vi "Shared Variable Creation.vi"() -> ()   [LabVIEW 2011]
uses:
  <vilib>/lvdsc/NI_DSC.lvlib
panel:
  out "error out 4":errorcluster
  out "error out 3":errorcluster
  out "error out 2":errorcluster
  out "error out":errorcluster
  out "process name out":string
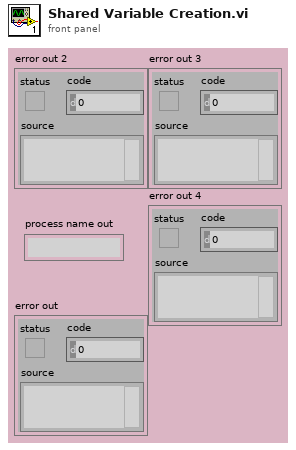
[diagram p1: front panel]
types:
  T1 = enum32{"u32BitField", "bool", "double", "string", "int8", "uint8", "int16", "uint16", "int32", "uint32", "int64", "uint64", "single", "double waveform", "int16 waveform", "array of boolean", "array of int8", "array of uint8", "array of int16", "array of uint16", "array of int32", "array of uint32", "array of int64", "array of uint64", "array of single", "array of double", "array of double waveform", "array of int16 waveform", "array of string", "variant", "timestamp", "fixed point", "custom"}
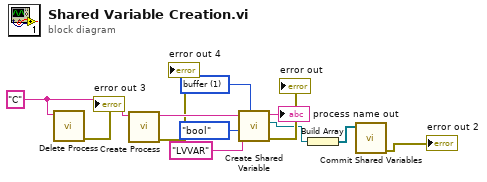
[diagram p0: block diagram]
diagram:
  w12 = u16 1 items=["commit", "buffer"] ("set mode")
  w4 = "C" ("process name")
  n1 = call <vilib>:"Delete Process.vi"("process name"=w4) -> ("error out"=→"error out 3":errorcluster)  [unwired: 1 in, 9 out]
  n2 = call <vilib>:"Create Process.vi"("process name"=w4) -> ("error out"=→"error out 4":errorcluster, "process name out"=w3:string)  [unwired: 5 in, 4 out]
  n3 = call <vilib>:"Create Shared Variable.vi"("set mode"=w12, "data type"=T1."bool", "shared variable name"="LVVAR", "process name"=w3) -> ("error out"=→"error out":errorcluster, "shared variable"=w7:refnum<k21>, "process name out"=→"process name out":string)  [unwired: 5 in]
  n4 = Build Array(w7) -> (w6:refnum<k21>[])
  n5 = call <vilib>:"Commit Shared Variables.vi"("shared variables"=w6) -> ("error out"=→"error out 2":errorcluster)  [unwired: 9 in, 1 out]
